vi "PhotonTargetModel_New_AprilTag16h5.vi"() -> (3 "PhotonTargetModel":T1 {"Vertices"."Z" format="%14.3f"; "Vertices"."Y" format="%14.3f"; "Vertices"."X" format="%14.3f"})   [LabVIEW 2019, in "PhotonVisionLib.lvlib"]
doc: "Create target model for 16h5 April Tag"
uses:
  PhotonVisionLib.lvlib
  TypeDef/PhotonTargetModel.ctl
  <vilib>/Rock Robotics/WPI/ThirdParty/JAS_Junk/TrajLib/TypeDef/TRANSLATION3D.ctl
  <vilib>/Rock Robotics/WPI/ThirdParty/JAS_Junk/TrajLib/VI/Translation3d_Create.vi
  PhotonTargetModel_New.vi
  <vilib>/Rock Robotics/WPI/ThirdParty/JAS_Junk/TrajLib/Trajectory_Library.lvlib
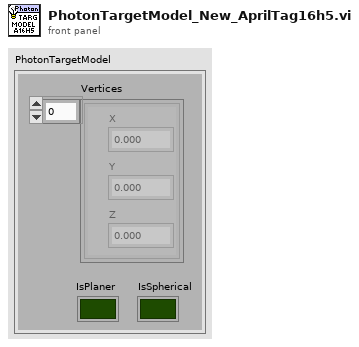
[diagram p1: front panel]
types:
  T1 = typedef "PhotonVisionLib.lvlib/PhotonTargetModel.ctl" = cluster{"Vertices":T2[], "IsPlaner":bool, "IsSpherical":bool}
  T2 = typedef "Trajectory_Library.lvlib/TRANSLATION3D.ctl" = cluster{"X":dbl, "Y":dbl, "Z":dbl}
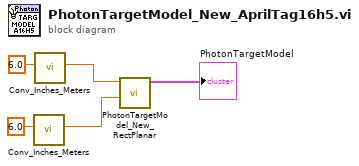
[diagram p0: block diagram]
diagram:
  n1 = call <vilib>:"Conv_Inches_Meters.vi"("INCH"=6.0) -> ("Meters"=w1:dbl)  [unwired: 10 in]
  n2 = call <vilib>:"Conv_Inches_Meters.vi"("INCH"=6.0) -> ("Meters"=w2:dbl)  [unwired: 10 in]
  n3 = call "PhotonTargetModel_New_RectPlanar.vi"("Height Meters"=w1, "Width Meters"=w2) -> ("PhotonTargetModel"=→"PhotonTargetModel":T1)  [unwired: 9 in]
